vi "random_array_2D.vi"(10 "x":i32=128, 11 "y":i32=128) -> (2 "array":i16[][](array[numeric]))   [LabVIEW 2015, in "daq_simulate.lvlib"]
uses:
  daq_simulate.lvlib
panel:
  in  "stability":dbl=3.0 format="%#_13g"
  in  "noise":dbl=0.15 format="%#_13g"
  in  "x0":i32=64
  in  "sigma":dbl=8.0
  in  "y0":i32=64
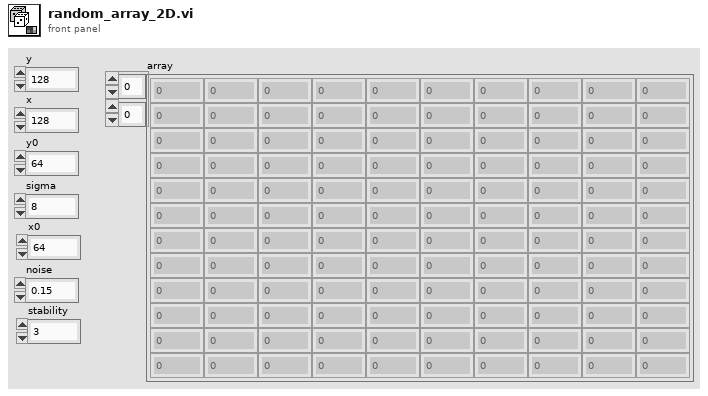
[diagram p1: front panel]
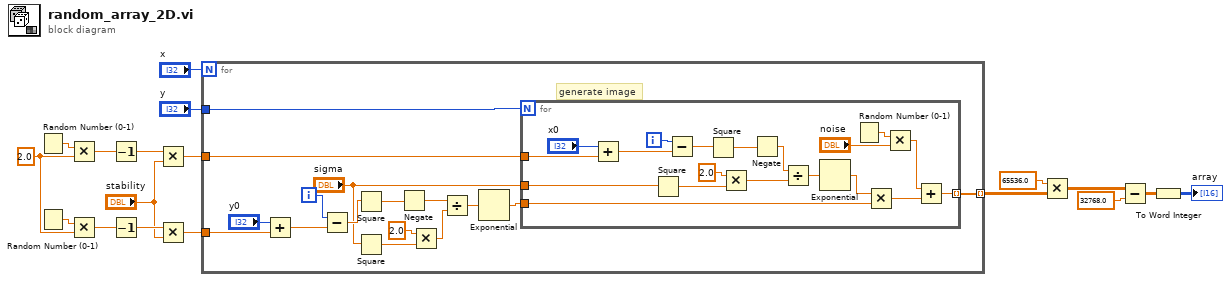
[diagram p0: block diagram]
diagram:
  w8 = 2.0 ("y")
  n1 = Random Number (0-1)() -> (number: 0 to 1=w10:dbl)
  n2 = Random Number (0-1)() -> (number: 0 to 1=w9:dbl)
  n3 = Multiply(x=w10, y=w8) -> (x*y=w7:dbl)
  n4 = Multiply(x=w9, y=w8) -> (x*y=w6:dbl)
  n5 = Decrement(x=w7) -> (x-1=w5:dbl)
  n6 = Decrement(x=w6) -> (x-1=w4:dbl)
  n7 = Multiply(x=w5, y="stability") -> (x*y=w2:dbl)
  n8 = Multiply(x=w4, y="stability") -> (x*y=w1:dbl)
  n9 = for {
    N: "x" -> [_]
    tunnel: [w34] -> w12 mode=indexing
    tunnel: "y" -> [w33]
    tunnel: w2 -> [w22]
    tunnel: w1 -> [w20]
    i -> [w32]
    # "generate image"
    n10 = Add(x="y0", y=w20) -> (x+y=w19:dbl)
    n11 = Subtract(x=w32, y=w19) -> (x-y=w31:dbl)
    n12 = Square(x=w31) -> (x^2=w30:dbl)
    n13 = Square(x="sigma") -> (x^2=w27:dbl)
    n14 = Negate(x=w30) -> (-x=w29:dbl)
    n15 = Multiply(x=2.0, y=w27) -> (x*y=w26:dbl)
    n16 = Divide(x=w29, y=w26) -> (x/y=w25:dbl)
    n17 = Exponential(1:w25) -> (0:w24:dbl)
    n18 = for {
      N: w33 -> [_]
      tunnel: [w40] -> w34 mode=indexing
      tunnel: w24 -> [w47]
      tunnel: "sigma" -> [w45]
      tunnel: w22 -> [w36]
      i -> [w44]
      n19 = Add(x="x0", y=w36) -> (x+y=w35:dbl)
      n20 = Square(x=w45) -> (x^2=w50:dbl)
      n21 = Subtract(x=w44, y=w35) -> (x-y=w43:dbl)
      n22 = Square(x=w43) -> (x^2=w53:dbl)
      n23 = Multiply(x=2.0, y=w50) -> (x*y=w49:dbl)
      n24 = Negate(x=w53) -> (-x=w52:dbl)
      n25 = Divide(x=w52, y=w49) -> (x/y=w48:dbl)
      n26 = Exponential(1:w48) -> (0:w46:dbl)
      n27 = Random Number (0-1)() -> (number: 0 to 1=w42:dbl)
      n28 = Multiply(x=w46, y=w47) -> (x*y=w39:dbl)
      n29 = Multiply(x=w42, y="noise") -> (x*y=w38:dbl)
      n30 = Add(x=w38, y=w39) -> (x+y=w40:dbl)
    }
  }
  n31 = Multiply(x=65536.0, y=w12) -> (x*y=w14:dbl[][])
  n32 = Subtract(x=w14, y=32768.0) -> (x-y=w11:dbl[][])
  n33 = To Word Integer(number=w11) -> (16bit integer=→"array":i16[][])
